vi "New Data.vi"(8 "error in (no error)":errorcluster, 10 "New Data":T1, 11 "Data Logger Module in":refnum<class "Data Logger DBL Module.lvclass">) -> (0 "error out":errorcluster, 2 "Split":bool, 3 "Data Logger Module out":refnum<class "Data Logger DBL Module.lvclass">)   [LabVIEW 2020, in "VolatusData.lvlib" / "Data Logger DBL Module.lvclass"]
uses:
  Data Logger DBL Module.lvclass
  New Data.ctl
  Data Logger DBL Module.lvclass/Data Logger DBL Module.ctl
  lv-vecto/Vecto/Double to Relative ns.vi
  lv-vecto/Vecto/Timestamp to Unix ns.vi
  VolatusData.lvlib
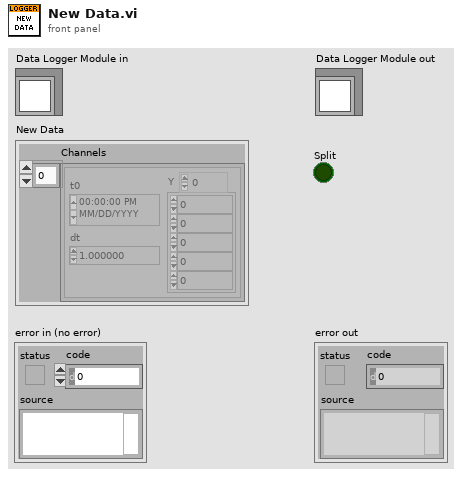
[diagram p1: front panel]
types:
  T1 = typedef "VolatusData.lvlib/New Data.ctl" = cluster{"Channels":waveform(dbl)[]}
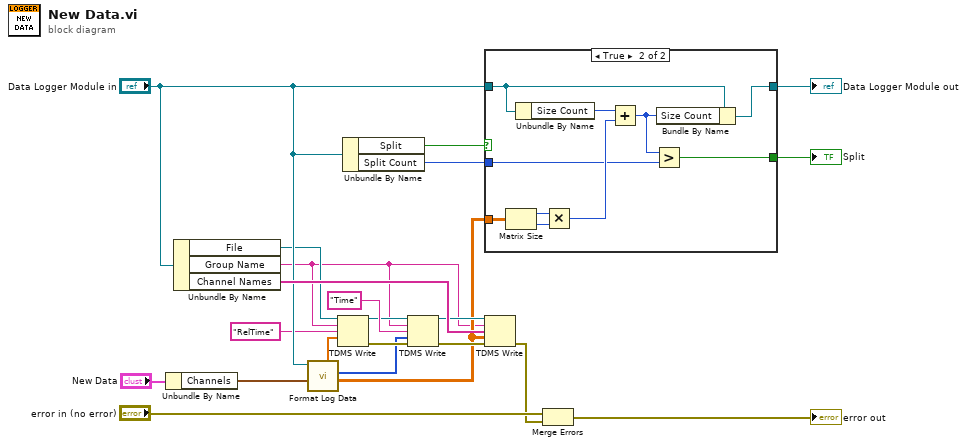
[diagram p0: block diagram]
diagram:
  n1 = Unbundle By Name("New Data") -> ("Channels"=w16:waveform(dbl)[])
  n2 = Unbundle By Name("Data Logger Module in") -> ("File"=w4:refnum<k34>, "Group Name"=w3:string, "Channel Names"=w15:string[])
  n3 = call "Format Log Data.vi"("Channels"=w16, "Data Logger Module in"="Data Logger Module in") -> ("Data"=w9:dbl[][], "Time"=w14:i64[], "Relative Time"=w1:dbl[])  [unwired: 5 in, 2 out]
  n4 = TDMS Write(0:w4, 5:w3, 7:"RelTime", 9:w1) -> (4:w5:refnum<k34>, 15:w22:errorcluster)  [unwired: 2 in, 2 out]
  n5 = Unbundle By Name("Data Logger Module in") -> ("Split"=w10:bool, "Split Count"=w8:i32)
  n6 = TDMS Write(0:w5, 5:w3, 7:"Time", 9:w14, 11:w22) -> (4:w12:refnum<k34>, 15:w21:errorcluster)  [unwired: 1 in, 2 out]
  n7 = case shown="True" w10 {
    tunnel: "Data Logger Module in" -> [w23 w28]
    tunnel: w9 -> [_ w31]
    tunnel: w8 -> [_ w25]
    tunnel: [w23 w27] -> w7
    tunnel: [_ w24] -> w6
    frame False {
    }
    frame True {
      n8 = Matrix Size(0:w31) -> (1:w33:i32, 2:w32:i32)
      n9 = Unbundle By Name(w28) -> ("Size Count"=w30:i32)
      n10 = Multiply(x=w33, y=w32) -> (x*y=w29:i32)
      n11 = Add(x=w30, y=w29) -> (x+y=w26:i32)
      n12 = Greater?(x=w26, y=w25) -> (0:w24:bool)
      n13 = Bundle By Name(cluster=w28, "Size Count"=w26) -> (w27:refnum<class "Data Logger DBL Module.lvclass">)
    }
  }
  "Data Logger Module out" <- w7
  "Split" <- w6
  n14 = TDMS Write(0:w12, 5:w3, 7:w15, 9:w9, 11:w21) -> (15:w17:errorcluster)  [unwired: 1 in, 3 out]
  n15 = Merge Errors("error in (no error)", w17) -> (→"error out":errorcluster)
